vi "Test.vi"() -> ()   [LabVIEW 2014]
doc: "This VI is called when test mode begins, and will automatically be terminated when it ends. You can add manual or automatic tests and invoke them from the dashboard."
uses:
  <vilib>/Rock Robotics/WPI/CAN/TalonSRX/WPI_CANTalonSRX_APIFeedbackSelect.ctl
  <vilib>/Rock Robotics/WPI/MotorControl/WPI_MotorControlOpenCANTalonSRX.vi
panel:
  out "Analog In":dbl
  out "Sensor Position":dbl
  in  "disable the motor":bool
  in  "Feedback Reference":T1
  in  "Set Ref":bool
  in  "enable the motor":bool
  in  "Device Number (set before running)":u8
  in  "close the motor and stop":bool
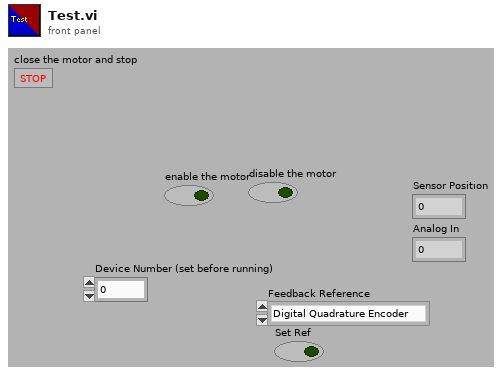
[diagram p1: front panel]
types:
  T1 = typedef "WPI_CANTalonSRX_APIFeedbackSelect.ctl" = enum16{"Digital Quadrature Encoder", "Analog Potentiometer", "Analog Encoder"}
  T2 = typedef "WPI_MotorControlDeviceRef.ctl" = cluster{"DeviceStatus":errorcluster, "Type":T3, "PWM":cluster{"Controller":T4, "PWM Channel":T5, "DeadBand":T6}, "CAN":cluster{"Device Number":u8, "Control Mode":T7, "Semaphore":T8, "Max Vout":dbl, "TalonSRX Control Mode":T9}, "Invert":bool, "TransformRef":T10, "InvTransformRef":T10}
  T3 = typedef "WPI_MotorControlType.ctl" = enum16{"PWM", "CAN", "CANTalonSRX"}
  T4 = typedef "FPGA_TypedefDigitalModule.ctl" = enum16{"Controller 1"}
  T5 = typedef "FPGA_DIOPWMChannel.ctl" = enum8{"PWM 0", "PWM 1", "PWM 2", "PWM 3", "PWM 4", "PWM 5", "PWM 6", "PWM 7", "PWM 8", "PWM 9", "PWM MXP 0", "PWM MXP 1", "PWM MXP 2", "PWM MXP 3", "PWM MXP 4", "PWM MXP 5", "PWM MXP 6", "PWM MXP 7", "PWM MXP 8", "PWM MXP 9", "Invalid"}
  T6 = typedef "WPI_PWMDeadband.ctl" = cluster{"Name":string, "maxPositivePwm":i32, "minPositivePwm":i32, "centerPwm":i32, "maxNegativePwm":i32, "minNegativePwm":i32, "angularRange":u16}
  T7 = typedef "WPI_CANJaguar_ControlMode.ctl" = enum8{"Percent VBus", "Current", "Speed", "Position", "Voltage"}
  T8 = typedef "Semaphore RefNum" = refnum<k1>
  T9 = typedef "WPI_CANTalonSRX_APIControlMode.ctl" = enum8{"Percent VBus", "Speed", "Position", "Slave", "Unchanged / Invalid"}
  T10 = typedef "WPI_PWMTransform_ConPane.ctl" = refnum<vi>
  T11 = typedef "WPI_CANTalonSRX_GlobalStatus.ctl" = cluster{"Applied Throttle":dbl, "Module Enabled":bool, "CAN Error":errorcluster, "Closed Loop Error":dbl, "Forward Limit Switch Closed":bool, "Reverse Limit Switch Closed":bool, "Sensor Position":dbl, "Sensor Velocity":dbl, "Current":dbl, "Sticky Fault - Over Temp":bool, "Sticky Fault - Under Voltage":bool, "Sticky Fault - Forward Limit":bool, "Sticky Fault - Reverse Limit":bool, "Sticky Fault - Forward Soft Limit":bool, "Sticky Fault - Reverse Soft Limit":bool, "Brake is Enabled":bool, "Encoder Position":dbl, "Encoder Velocity":dbl, "Encoder Index Count":dbl, "Encoder A Pin State":bool, "Encoder B Pin State":bool, "Encoder Index Pin State":bool, "Analog In":dbl, "Analog In Velocity":dbl, "Temperature (C)":dbl, "Battery Voltage":dbl}
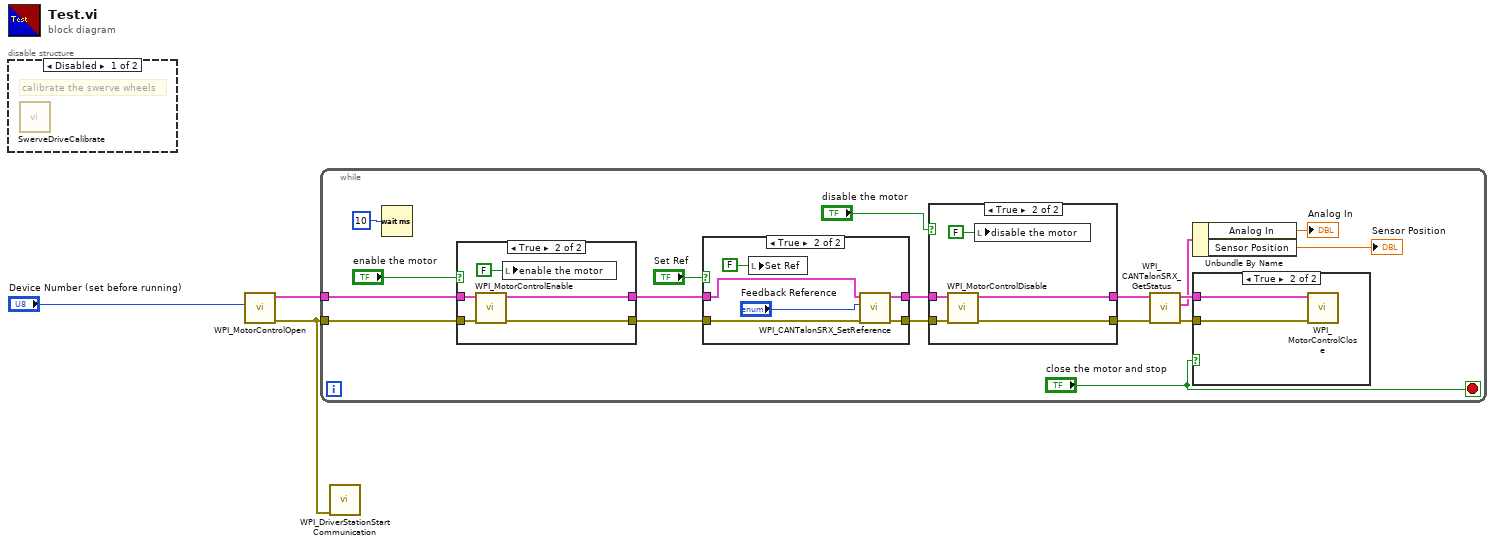
[diagram p0: block diagram]
diagram:
  n1 = disable-structure shown="Disabled" {
    frame Disabled {
      # "calibrate the swerve wheels"
      n2 = call "SwerveDriveCalibrate.vi"() -> ()  [unwired: 12 in]
    }
    frame Enabled {
    }
  }
  n3 = call-poly <vilib>:"WPI_MotorControlOpen.vi"("Device Number"="Device Number (set before running)") -> ("error out"=w1:errorcluster, "MotorControlDeviceRef"=w2:T2)  [unwired: 9 in]
  n4 = while {
    tunnel: w2 -> [w19]
    tunnel: w1 -> [w18]
    stop <- "close the motor and stop" stop-if-true
    n5 = Wait (ms)(milliseconds to wait=u32 10) -> ()  [unwired: 1 out]
    n6 = case shown="True" "enable the motor" {
      tunnel: w19 -> [w40 w45]
      tunnel: w18 -> [w39 w44]
      tunnel: [w40 w43] -> w15
      tunnel: [w39 w42] -> w14
      frame False {
      }
      frame True {
        n7 = call <vilib>:"WPI_MotorControlEnable.vi"("error in (no error)"=w44, "CAN Jaguar Ref"=w45) -> ("error out"=w42:errorcluster, "CAN Jaguar Ref Out"=w43:T2)  [unwired: 8 in]
        n8 = local write "enable the motor"(FALSE ("enable the motor")) -> ()
      }
    }
    n9 = case shown="True" "Set Ref" {
      tunnel: w15 -> [w32 w37]
      tunnel: w14 -> [w31 w36]
      tunnel: [w32 w34] -> w12
      tunnel: [w31 w33] -> w11
      frame False {
      }
      frame True {
        n10 = local write "Set Ref"(FALSE ("Set Ref")) -> ()
        n11 = call <vilib>:"WPI_CANTalonSRX_SetReference.vi"("error in (no error)"=w36, "Feedback Reference"="Feedback Reference", "CAN Talon SRX Ref"=w37) -> ("error out"=w33:errorcluster, "CAN Talon SRX Ref Out"=w34:T2)  [unwired: 7 in]
      }
    }
    n12 = case shown="True" "disable the motor" {
      tunnel: w12 -> [w25 w29]
      tunnel: w11 -> [w24 w28]
      tunnel: [w25 w27] -> w10
      tunnel: [w24 w26] -> w8
      frame False {
      }
      frame True {
        n13 = call <vilib>:"WPI_MotorControlDisable.vi"("error in (no error)"=w28, "MotorControlDevRef"=w29) -> ("error out"=w26:errorcluster, "MotorControlDevRef"=w27:T2)  [unwired: 8 in]
        n14 = local write "disable the motor"(FALSE ("disable the motor")) -> ()
      }
    }
    n15 = call <vilib>:"WPI_CANTalonSRX_GetStatus.vi"("error in (no error)"=w8, "CAN Talon SRX Ref"=w10) -> ("error out"=w7:errorcluster, "Talon SRX Status"=w6:T11, "CAN Talon SRX Ref Out"=w9:T2)  [unwired: 7 in]
    n16 = Unbundle By Name(w6) -> ("Analog In"=→"Analog In":dbl, "Sensor Position"=→"Sensor Position":dbl)
    n17 = case shown="True" "close the motor and stop" {
      tunnel: w9 -> [_ w23]
      tunnel: w7 -> [_ w22]
      frame False {
      }
      frame True {
        n18 = call <vilib>:"WPI_MotorControlClose.vi"("error in (no error)"=w22, "MotorControlDevRef"=w23) -> ()  [unwired: 9 in, 1 out]
      }
    }
  }
  n19 = call <vilib>:"WPI_DriverStationStart Communication.vi"("error in (no error)"=w1) -> ()  [unwired: 11 in]
